vi "PID.vi"(1 "Present Value":dbl=15.0 format="%.2f", 2 "Previous Control Sum":dbl format="%.2f", 3 "Setpoint":dbl=15.0 format="%.2f") -> (0 "Dem Output":dbl format="%.2f")   [LabVIEW 2010]
uses:
  <vilib>/Analysis/NI_AALPro.lvlib
panel:
  in  "O/P deadband":dbl=1.0 format="%.2f"
  in  "Kp Deadband":dbl format="%.2f"
  in  "Derivative History":i32=20
  out "deadbanded error":dbl format="%.2f"
  in  "P":bool=TRUE
  in  "D":bool=TRUE
  in  "I":bool=TRUE
  out "Waveform Chart":T1(graph)
  in  "Manual Demand":dbl min=0.0 max=100.0 format="%.2f"
  in  "Manual Override":bool
  out "Control Sum":dbl format="%.2f"
  out "Derivative Term":dbl format="%.2f"
  out "Integral Term":dbl format="%.2f"
  out "error differential":dbl format="%.5f"
  out "error integral":dbl format="%.2f"
  out "Proportional Term":dbl format="%.2f"
  in  "Kd":dbl=50.0 format="%.2f"
  in  "Ki":dbl=10.0 format="%.2f"
  in  "Kp":dbl=5.0 format="%.2f"
  out "error":dbl format="%.2f"
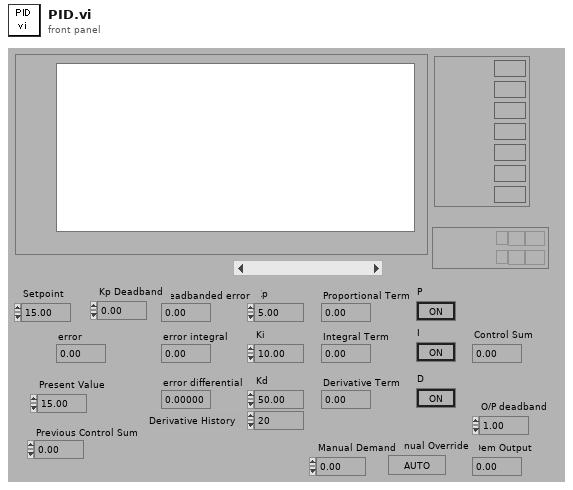
[diagram p1: front panel]
types:
  T1 = cluster{"Setpoint":dbl, "Present Value":dbl, "Proportional Term":dbl, "Integral Term":dbl, "Derivative Term":dbl, "Control Sum":dbl, "Dem Output":dbl}
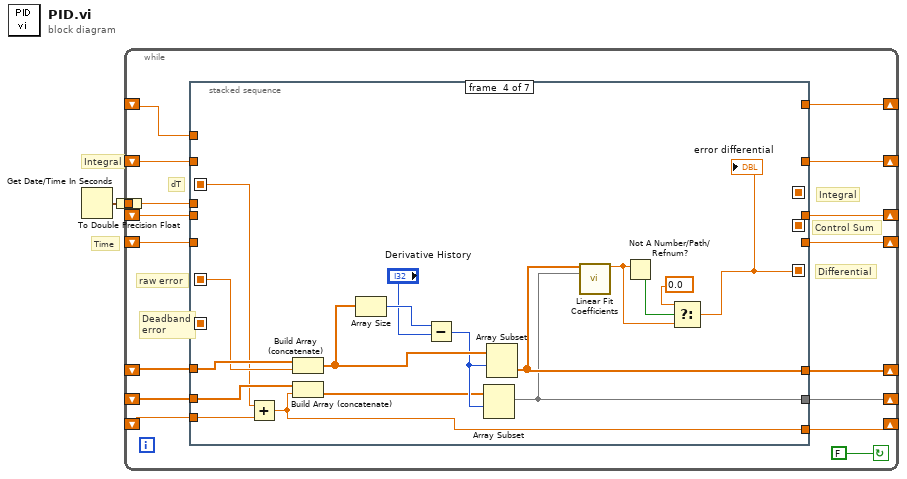
[diagram p0: block diagram]
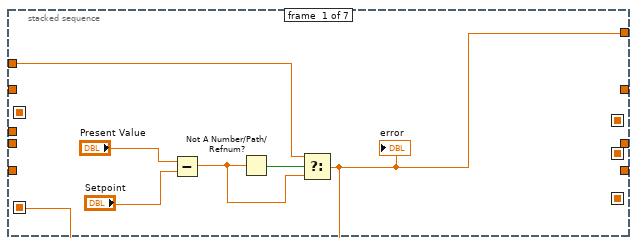
[diagram p2: hidden frame]
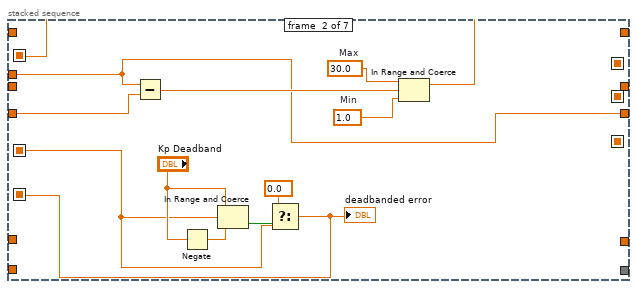
[diagram p3: hidden frame]
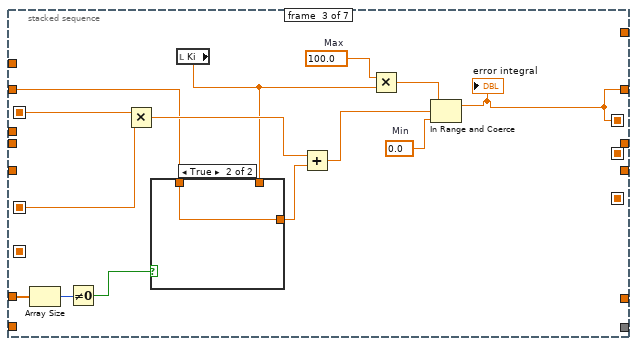
[diagram p4: hidden frame]
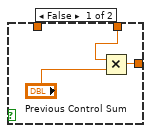
[diagram p5: hidden frame]
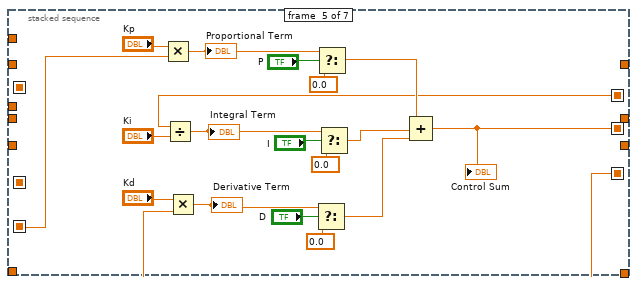
[diagram p6: hidden frame]
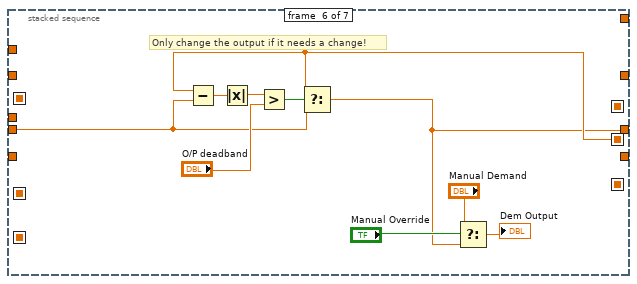
[diagram p7: hidden frame]
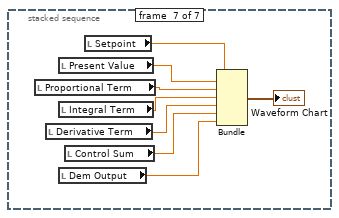
[diagram p8: hidden frame]
diagram:
  # "Integral"
  # "Time"
  n1 = Get Date/Time In Seconds() -> (seconds since 1Jan1904=w1:timestamp)
  n2 = To Double Precision Float(number=w1) -> (double precision float=w2:dbl)
  n3 = while {
    shift-left: _ -> [w5]
    shift-right: [w4] -> _
    shift-left: _ -> [w7]
    shift-right: [w6] -> _
    shift-left: _ -> [w9]
    shift-right: [w8] -> _
    tunnel: w2 -> [w14]
    shift-left: _ -> [w11]
    shift-right: [w10] -> _
    shift-left: _ -> [w13]
    shift-right: [w12] -> _
    shift-left: _ -> [w15]
    shift-right: [w16] -> _
    shift-left: _ -> [w18]
    shift-right: [w17] -> _
    stop <- FALSE continue-if-true
    # "Control Sum"
    # "raw error"
    # "Differential"
    # "Integral"
    # "Deadband\nerror"
    # "dT"
    n4 = stacked-sequence {
      seq-local: [_ w25 _ _ _ _ _] -> [_ _ w50 w57 _ _ _]
      seq-local: [_ w34 _ _ _ _ _] -> [_ _ _ _ w75 _ _]
      seq-local: [_ _ _ w62 _ _ _] -> [_ _ _ _ w74 _ _]
      seq-local: [_ _ w37 _ _ _ _] -> [_ _ _ _ w73 _ _]
      seq-local: [w19 _ _ _ _ _ _] -> [_ w26 w45 w63 _ _ _]
      seq-local: [_ _ _ _ w78 _ _] -> [_ _ _ _ _ w94 _]
      tunnel: w18 -> [_ w31 _ _ _ _ _]
      tunnel: [_ w29 _ _ _ _ _] -> w17
      tunnel: [_ _ w37 _ _ _ _] -> w16
      tunnel: w15 -> [_ _ w39 _ _ _ _]
      tunnel: w14 -> [_ w29 _ _ _ _ _]
      tunnel: w13 -> [_ _ w44 w71 _ _ _]
      tunnel: [_ _ _ w64 _ _ _] -> w12
      tunnel: w11 -> [_ _ _ w70 _ _ _]
      tunnel: [_ _ _ w61 _ _ _] -> w10
      tunnel: w9 -> [_ _ _ _ _ w92 _]
      tunnel: [_ _ _ _ _ w91 _] -> w8
      tunnel: w7 -> [_ _ _ w56 _ _ _]
      tunnel: [_ _ _ w55 _ _ _] -> w6
      tunnel: w5 -> [w21 _ _ _ _ _ _]
      tunnel: [w19 _ _ _ _ _ _] -> w4
      frame #0 {
        n5 = Subtract(x="Present Value", y="Setpoint") -> (x-y=w20:dbl)
        n6 = Not A Number/Path/Refnum?(number/path/refnum=w20) -> (NaN/Path/Refnum?=w22:bool)
        n7 = Select(t=w21, s=w22, f=w20) -> (s? t:f=w19:dbl)
        "error" <- w19
      }
      frame #1 {
        w32 = 1.0  # Min
        w33 = 30.0  # Max
        n8 = Subtract(x=w29, y=w31) -> (x-y=w30:dbl)
        n9 = Negate(x="Kp Deadband") -> (-x=w28:dbl)
        n10 = In Range and Coerce(upper limit="Kp Deadband", x=w26, lower limit=w28) -> (In Range?=w35:bool)  [unwired: 1 out]
        n11 = Select(t=0.0, s=w35, f=w26) -> (s? t:f=w34:dbl)
        "deadbanded error" <- w34
        n12 = In Range and Coerce(upper limit=w33, x=w30, lower limit=w32) -> (coerced(x)=w25:dbl)  [unwired: 1 out]
      }
      frame #2 {
        w49 = 0.0  # Min
        w48 = 100.0  # Max
        n13 = Array Size(array=w44) -> (size(s)=w43:i32)
        n14 = Not Equal To 0?(x=w43) -> (x != 0?=w41:bool)
        n15 = Multiply(x=w50, y=w45) -> (x*y=w42:dbl)
        n16 = local read "Ki"() -> (w38:dbl)
        n17 = case shown="True" w41 {
          tunnel: [w51 w54] -> w40
          tunnel: w39 -> [_ w54]
          tunnel: w38 -> [w53 _]
          frame False {
            n18 = Multiply(x=w53, y="Previous Control Sum") -> (x*y=w51:dbl)
          }
          frame True {
          }
        }
        n19 = Add(x=w42, y=w40) -> (x+y=w46:dbl)
        n20 = Multiply(x=w48, y=w38) -> (x*y=w47:dbl)
        n21 = In Range and Coerce(upper limit=w47, x=w46, lower limit=w49) -> (coerced(x)=w37:dbl)  [unwired: 1 out]
        "error integral" <- w37
      }
      frame #3 {
        n22 = Add(x=w57, y=w56) -> (x+y=w55:dbl)
        n23 = Build Array (concatenate)(w71, w63) -> (w67:dbl[])
        n24 = Build Array (concatenate)(w70, w55) -> (w65:dbl[])
        n25 = Array Size(array=w67) -> (size(s)=w69:i32)
        n26 = Subtract(x=w69, y="Derivative History") -> (x-y=w66:i32)
        n27 = Array Subset(array=w65, index=w66) -> (w61:dbl[])  [unwired: 1 in]
        n28 = Array Subset(array=w67, index=w66) -> (w64:dbl[])  [unwired: 1 in]
        n29 = call <vilib>:"Linear Fit Coefficients.vi"("Y"=w64, "X"=w61) -> ("slope"=w58:dbl)  [unwired: 3 in, 10 out]
        n30 = Not A Number/Path/Refnum?(number/path/refnum=w58) -> (NaN/Path/Refnum?=w60:bool)
        n31 = Select(t=0.0 ("f"), s=w60, f=w58) -> (s? t:f=w62:dbl)
        "error differential" <- w62
      }
      frame #4 {
        n32 = Multiply(x="Kp", y=w75) -> (x*y=w88:dbl)
        "Proportional Term" <- w88
        n33 = Divide(x=w73, y="Ki") -> (x/y=w79:dbl)
        "Integral Term" <- w79
        n34 = Multiply(x="Kd", y=w74) -> (x*y=w80:dbl)
        "Derivative Term" <- w80
        n35 = Select(t=w80, s="D", f=0.0) -> (s? t:f=w82:dbl)
        n36 = Select(t=w88, s="P", f=0.0) -> (s? t:f=w89:dbl)
        n37 = Select(t=w79, s="I", f=0.0) -> (s? t:f=w81:dbl)
        n38 = Compound Arithmetic op=ADD(w89, w81, w82) -> (w78:dbl)
        "Control Sum" <- w78
      }
      frame #5 {
        # "Only change the output if it needs a change!"
        n39 = Subtract(x=w94, y=w92) -> (x-y=w97:dbl)
        n40 = Absolute Value(x=w97) -> (abs(x)=w96:dbl)
        n41 = Greater?(x=w96, y="O/P deadband") -> (0:w95:bool)
        n42 = Select(t=w94, s=w95, f=w92) -> (s? t:f=w91:dbl)
        n43 = Select(t="Manual Demand", s="Manual Override", f=w91) -> (s? t:f=→"Dem Output":dbl)
      }
      frame #6 {
        n44 = local read "Proportional Term"() -> (w104:dbl)
        n45 = local read "Derivative Term"() -> (w106:dbl)
        n46 = local read "Present Value"() -> (w103:dbl)
        n47 = local read "Integral Term"() -> (w105:dbl)
        n48 = local read "Dem Output"() -> (w108:dbl)
        n49 = local read "Control Sum"() -> (w107:dbl)
        n50 = local read "Setpoint"() -> (w102:dbl)
        n51 = Bundle("Setpoint"=w102, "Present Value"=w103, "Proportional Term"=w104, "Integral Term"=w105, "Derivative Term"=w106, "Control Sum"=w107, "Dem Output"=w108) -> (→"Waveform Chart":T1)  [unwired: 1 out]
      }
    }
  }
